vi "CoboltLaser_ComPortWrite.vi"(0 "ComPort":refnum<visa-resource-name>, 1 "Command":string, 2 "Data":string, 5 "error in (no error)":errorcluster) -> (14 "ComPortOut":refnum<visa-resource-name>, 19 "error out":errorcluster)   [LabVIEW 2019]
doc: "Use this template to build a VI to use as a subVI."
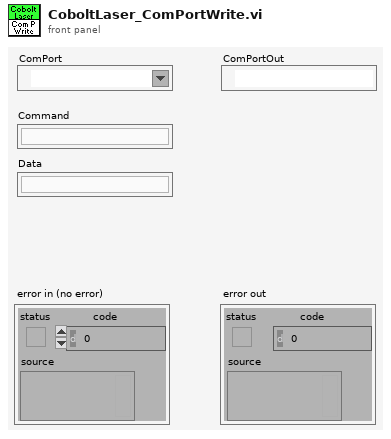
[diagram p1: front panel]
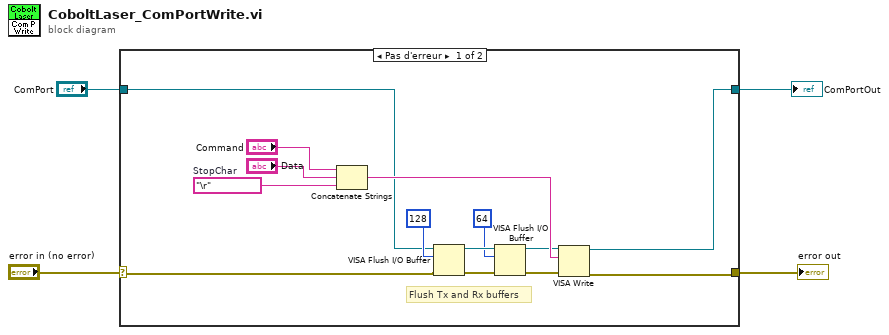
[diagram p0: block diagram]
diagram:
  n1 = case shown="Pas d'erreur" "error in (no error)" {
    selector: "error in (no error)" -> [w13 w20]
    tunnel: [w5 w20] -> w3
    tunnel: "ComPort" -> [w7 w19]
    tunnel: [w6 w19] -> w1
    frame No Error {
      w8 = "\r"  # StopChar
      # "Flush Tx and Rx buffers"
      n2 = Concatenate Strings("Command", "Data", w8) -> (w18:string)
      n3 = VISA Flush I/O Buffer(VISA resource name=w7, mask (16)=u16 128, error in (no error)=w13) -> (VISA resource name out=w16:refnum<visa-resource-name>, error out=w17:errorcluster)
      n4 = VISA Flush I/O Buffer(VISA resource name=w16, mask (16)=u16 64, error in (no error)=w17) -> (VISA resource name out=w11:refnum<visa-resource-name>, error out=w12:errorcluster)
      n5 = VISA Write(VISA resource name=w11, write buffer=w18, error in (no error)=w12) -> (VISA resource name out=w6:refnum<visa-resource-name>, error out=w5:errorcluster)  [unwired: 1 out]
    }
    frame Error {
    }
  }
  "error out" <- w3
  "ComPortOut" <- w1
